vi "Add Password.vi"(8 "error in (no error)":errorcluster, 10 "Write Password":string, 11 "Master in":refnum<class "MASTER.lvclass">) -> (0 "error out":errorcluster, 3 "Master out":refnum<class "MASTER.lvclass">)   [LabVIEW 2014, in "Files Library.lvlib" / "Master.lvclass"]
uses:
  MASTER/MASTER.lvclass
  MASTER/MASTER.lvclass/MASTER.ctl
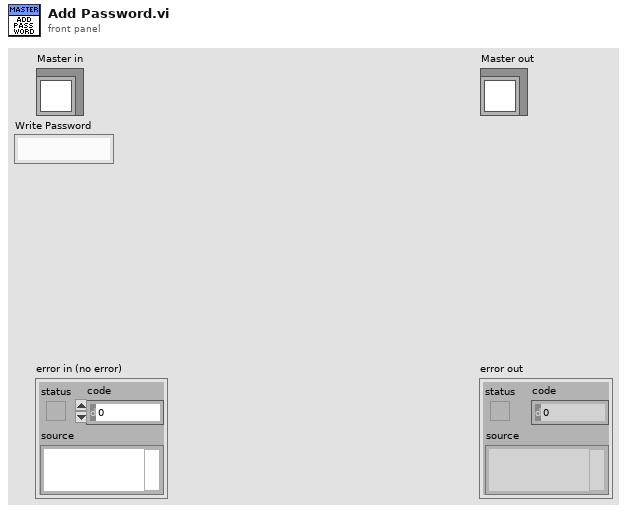
[diagram p1: front panel]
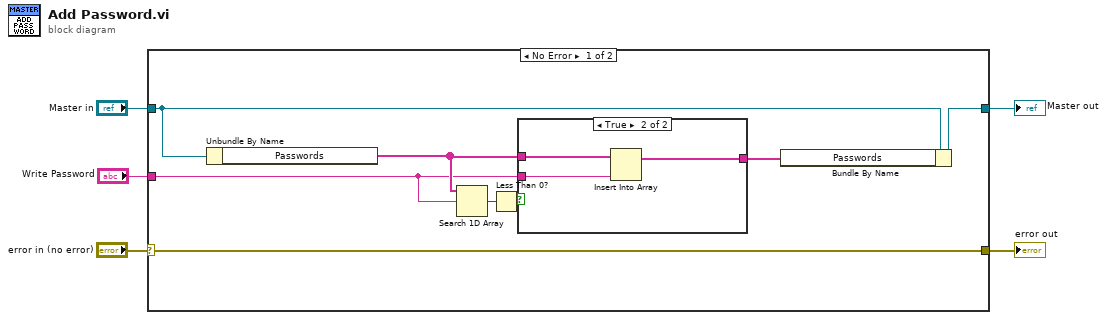
[diagram p0: block diagram]
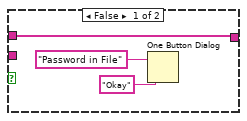
[diagram p2: hidden frame]
diagram:
  n1 = case shown="No Error" "error in (no error)" {
    selector: "error in (no error)" -> [w13 w21]
    tunnel: [w13 w21] -> w4
    tunnel: [w11 w20] -> w2
    tunnel: "Master in" -> [w12 w20]
    tunnel: "Write Password" -> [w6 _]
    frame No Error {
      n2 = Unbundle By Name(w12) -> ("Passwords"=w9:string[])
      n3 = Search 1D Array(1D array=w9, element=w6) -> (index of element=w8:i32)  [unwired: 1 in]
      n4 = Less Than 0?(x=w8) -> (x < 0?=w7:bool)
      n5 = case shown="True" w7 {
        tunnel: [w16 w19] -> w10
        tunnel: w9 -> [w16 w18]
        tunnel: w6 -> [_ w17]
        frame False {
          n6 = One Button Dialog(message="Password in File", button name ("OK")="Okay") -> ()  [unwired: 1 out]
        }
        frame True {
          n7 = Insert Into Array(array=w18, new element=w17) -> (w19:string[])  [unwired: 1 in]
        }
      }
      n8 = Bundle By Name(cluster=w12, "Passwords"=w10) -> (w11:refnum<class "MASTER.lvclass">)
    }
    frame Error {
    }
  }
  "error out" <- w4
  "Master out" <- w2
